vi "gentec-M-Link.VI Tree.vi"   [LabVIEW 2014, in "gentec-M-Link - Driver.lvlib"]
doc: "This is the instrument driver for the gentec M-Link Powermeter. The VI Tree displays all the user-callable VIs of the instrument driver in an organized table."
uses:
  gentec-M-Link - Driver.lvlib
  Driver/Type Defs/gentec-M-Link.Range.ctl
  Driver/Type Defs/gentec-M-Link.Measurement Mode.ctl
  Driver/Type Defs/gentec-M-Link.Trigger Polarity.ctl
  Driver/Type Defs/gentec-M-Link.Trigger Source.ctl
  Driver/Type Defs/gentec-M-Link.Queries with String Answers.ctl
  Driver/Type Defs/gentec-M-Link.Range Queries.ctl
  Driver/Type Defs/gentec-M-Link.Waveform Averages.ctl
panel:
  # "SEE DIAGRAM\nFOR VI TREE."
types:
  T1 = typedef "gentec-M-Link - Driver.lvlib/gentec-M-Link.Waveform Averages.ctl" = u16
  T2 = typedef "gentec-M-Link - Driver.lvlib/gentec-M-Link.Range Queries.ctl" = string
  T3 = typedef "gentec-M-Link - Driver.lvlib/gentec-M-Link.Queries with String Answers.ctl" = string
  T4 = typedef "gentec-M-Link - Driver.lvlib/gentec-M-Link.Trigger Source.ctl" = u16
  T5 = typedef "gentec-M-Link - Driver.lvlib/gentec-M-Link.Trigger Polarity.ctl" = u16
  T6 = typedef "gentec-M-Link - Driver.lvlib/gentec-M-Link.Measurement Mode.ctl" = u16
  T7 = typedef "gentec-M-Link - Driver.lvlib/gentec-M-Link.Range.ctl" = u16
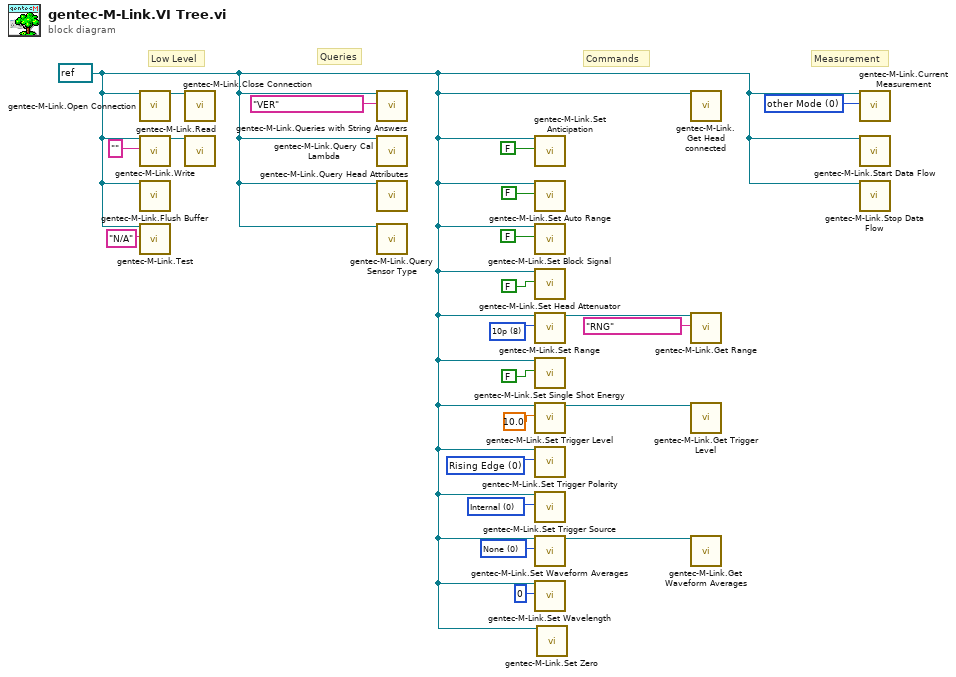
[diagram p0: block diagram]
diagram:
  w10 = T1 0 items=["None", "2", "4", "8", "16", "32", "64", "128"] ("Waveform Averages")
  w15 = T4 0 items=["Internal", "External"] ("Trigger Source")
  w16 = T5 0 items=["Rising Edge", "Falling Edge"] ("Trigger Polarity")
  w18 = T6 0 items=["other Mode", "Energymode"] ("Measurement")
  w19 = T7 8 items=["1f", "3f", "10f", "30f", "100f", "300f", "1p", "3p", "10p", "30p", "100p", "300p", "1n", "3n", "10n", "30n", "100n", "300n", "1u", "3u", "10u", "30u", "100u", "300u", "1m", "3m", "10m", "30m", "100m", "300m", "1", "3", "10", "30", "100", "300", "1K", "3K", "10K", "30K", "100K", "300K", "1M", "3M", "10M", "30M", "100M", "300M"] ("Range")
  w2 = refnum<visa-resource-name> refnum ("VISA resource In")
  # "Measurement"
  # "Commands"
  # "Queries"
  # "Low Level"
  n1 = call "gentec-M-Link.Open Connection.vi"("VISA resource (In)"=w2) -> ("VISA resource (Out)"=w6:refnum<visa-resource-name>)  [unwired: 17 in, 1 out]
  n2 = call "gentec-M-Link.Write.vi"("VISA resource (In)"=w2, "Data To Write"="") -> ("VISA resource (Out)"=w7:refnum<visa-resource-name>)  [unwired: 15 in, 2 out]
  n3 = call "gentec-M-Link.Flush Buffer.vi"("VISA resource(In)"=w2) -> ()  [unwired: 16 in, 3 out]
  n4 = call "gentec-M-Link.Test.vi"("VISA resource In"=w2, "Data to Write"="N/A") -> ()  [unwired: 14 in, 4 out]
  n5 = call "gentec-M-Link.Close Connection.vi"("VISA resource In"=w6) -> ()  [unwired: 18 in, 1 out]
  n6 = call "gentec-M-Link.Read.vi"("VISA resource (In)"=w7) -> ()  [unwired: 14 in, 5 out]
  n7 = call "gentec-M-Link.Queries with String Answers.vi"("VISA resource In"=w2, "Queries with String Answers"=T3 "VER") -> ()  [unwired: 14 in, 4 out]
  n8 = call "gentec-M-Link.Query Cal Lambda.vi"("VISA resource In"=w2) -> ()  [unwired: 14 in, 5 out]
  n9 = call "gentec-M-Link.Query Head Attributes.vi"("VISA resource In"=w2) -> ()  [unwired: 14 in, 5 out]
  n10 = call "gentec-M-Link.Query Sensor Type.vi"("VISA resource In"=w2) -> ()  [unwired: 14 in, 5 out]
  n11 = call "gentec-M-Link.Set Anticipation.vi"("VISA resource In"=w2, "Enable Anticipation"=FALSE) -> ()  [unwired: 13 in, 5 out]
  n12 = call "gentec-M-Link.Set Auto Range.vi"("VISA resource In"=w2, "Auto Range"=FALSE) -> ()  [unwired: 13 in, 5 out]
  n13 = call "gentec-M-Link.Set Block Signal.vi"("VISA resource In"=w2, "Block Signal"=FALSE) -> ()  [unwired: 16 in, 2 out]
  n14 = call "gentec-M-Link.Set Head Attenuator.vi"("VISA resource In"=w2, "Set Head Attenuator"=FALSE) -> ()  [unwired: 12 in, 6 out]
  n15 = call "gentec-M-Link.Set Range.vi"("VISA resource In"=w2, "Range"=w19) -> ("VISA resource Out"=w8:refnum<visa-resource-name>)  [unwired: 13 in, 4 out]
  n16 = call "gentec-M-Link.Set Single Shot Energy.vi"("VISA resource In"=w2, "Enable Single Shot Energy"=FALSE) -> ()  [unwired: 12 in, 6 out]
  n17 = call "gentec-M-Link.Set Trigger Level.vi"("VISA resource In"=w2, "Trigger Level [%]"=10.0) -> ("VISA resource Out"=w9:refnum<visa-resource-name>)  [unwired: 13 in, 4 out]
  n18 = call "gentec-M-Link.Set Trigger Polarity.vi"("VISA resource In"=w2, "Trigger Polarity"=w16) -> ()  [unwired: 13 in, 5 out]
  n19 = call "gentec-M-Link.Set Trigger Source.vi"("VISA resource In"=w2, "Trigger Source"=w15) -> ()  [unwired: 16 in, 2 out]
  n20 = call "gentec-M-Link.Set Waveform Averages.vi"("VISA resource In"=w2, "Waveform Averages"=w10) -> ("VISA resource Out"=w4:refnum<visa-resource-name>)  [unwired: 13 in, 4 out]
  n21 = call "gentec-M-Link.Set Wavelength.vi"("VISA resource In"=w2, "Lambda"=u16 0) -> ()  [unwired: 9 in, 9 out]
  n22 = call "gentec-M-Link.Set Zero.vi"("VISA resource (In)"=w2) -> ()  [unwired: 11 in, 8 out]
  n23 = call "gentec-M-Link.Get Head connected.vi"("VISA resource In"=w2) -> ()  [unwired: 14 in, 5 out]
  n24 = call "gentec-M-Link.Get Range.vi"("VISA resource In"=w8, "Range Queries"=T2 "RNG") -> ()  [unwired: 12 in, 6 out]
  n25 = call "gentec-M-Link.Get Trigger Level.vi"("VISA resource In"=w9) -> ()  [unwired: 13 in, 6 out]
  n26 = call "gentec-M-Link.Get Waveform Averages.vi"("VISA resource In"=w4) -> ()  [unwired: 14 in, 5 out]
  n27 = call "gentec-M-Link.Current Measurement.vi"("VISA resource In"=w2, "Measurement"=w18) -> ()  [unwired: 8 in, 10 out]
  n28 = call "gentec-M-Link.Start Data Flow.vi"("VISA resource In"=w2) -> ()  [unwired: 17 in, 2 out]
  n29 = call "gentec-M-Link.Stop Data Flow.vi"("VISA resource In"=w2) -> ()  [unwired: 14 in, 5 out]
